vi "UTF8 LV80.vi"() -> ()   [LabVIEW 2017]
panel:
  out "utf-8 text out":string
  out "text out":string
  in  "text":string
  in  "utf-8 text":string
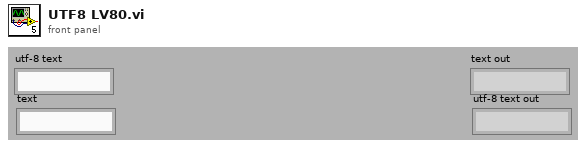
[diagram p1: front panel]
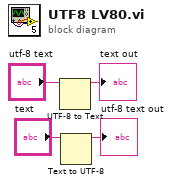
[diagram p0: block diagram]
diagram:
  n1 = UTF-8 to Text(11:"utf-8 text") -> (3:→"text out":string)  [unwired: 2 in, 1 out]
  n2 = Text to UTF-8(11:"text") -> (3:→"utf-8 text out":string)  [unwired: 2 in, 1 out]
